vi "WriteMultipleDataToImage.vi"(0 "Device in":refnum<class "Device.lvclass">, 5 "Image In":T1, 7 "Keys":string[](array[string]), 9 "Values":dbl[](array[numeric]), 11 "error in (no error)":errorcluster, 12 "precision (6)":i16) -> (4 "Device out":refnum<class "Device.lvclass">, 6 "Image Out":T1, 15 "error out":errorcluster)   [LabVIEW 2020, in "Device.lvlib" / "Device.lvclass"]
uses:
  Device.lvclass
  <vilib>/vision/Image Controls.llb/IMAQ Image.ctl
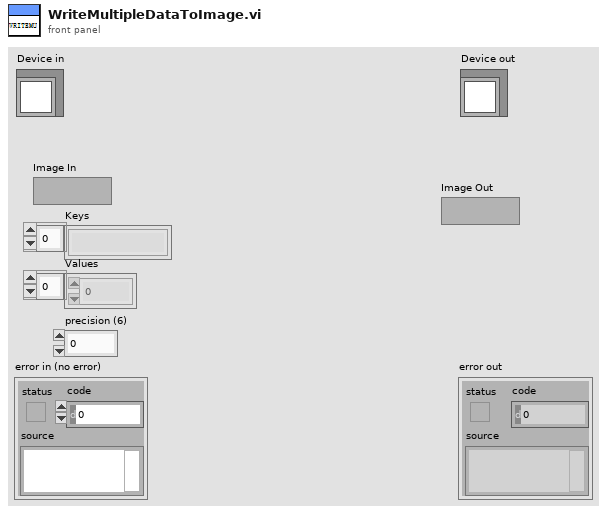
[diagram p1: front panel]
types:
  T1 = typedef "IMAQ Image.ctl" = refnum<image>
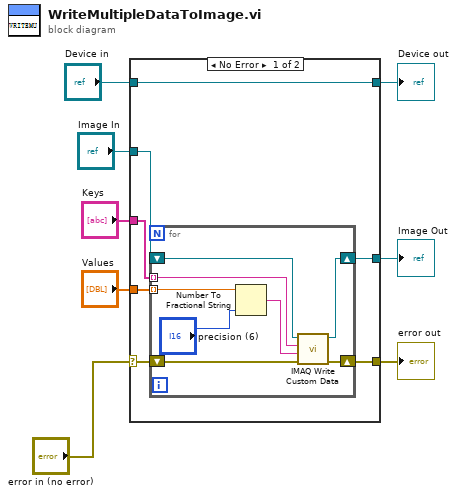
[diagram p0: block diagram]
diagram:
  n1 = case shown="No Error" "error in (no error)" {
    selector: "error in (no error)" -> [w14 w26]
    tunnel: [w13 w26] -> w7
    tunnel: [w15 w25] -> w5
    tunnel: "Device in" -> [w15 w25]
    tunnel: "Image In" -> [w12 w24]
    tunnel: "Values" -> [w9 _]
    tunnel: "Keys" -> [w10 _]
    tunnel: [w11 w24] -> w1
    frame No Error {
      n2 = for {
        tunnel: w10 -> [w18] mode=indexing
        tunnel: w9 -> [w17] mode=indexing
        shift-right: [w22] -> w13
        shift-left: w14 -> [w23]
        shift-right: [w20] -> w11
        shift-left: w12 -> [w21]
        n3 = Number To Fractional String(number=w17, precision (6)="precision (6)") -> (F-format string=w19:string)  [unwired: 2 in]
        n4 = call "IMAQ Write Custom Data"("error in (no error)"=w23, "Custom Data In"=w19, "Key"=w18, "Image"=w21) -> ("error out"=w22:errorcluster, "Image Out"=w20:T1)  [unwired: 6 in]
      }
    }
    frame Error {
    }
  }
  "error out" <- w7
  "Device out" <- w5
  "Image Out" <- w1
